vi "csm_lumikki_instron_creep_poller.vi"() -> ()   [LabVIEW 2009]
doc: "This is the sample data playback waveform and data logging example program. Sample data points are generated using MX Sample Data Array Generator.vi. You will need to replace this VI with your own code. New sample data is sent to the controller each time a status message is recieved from the controller that the next random buffer is running.\nThis program also shows you how to use Active X events. These are used to notify the program when a data buffer is ready for collection and when to load a new buffer of sample data points. Two separate event queues are used: one for data logging and the other for general status, such as when a sample data point buffer can be sent to the controller. Each event handler must run in parallel loops as execution passes to MX Handle Status Change Event.vi and MX Handle Data Ready Event.vi and will not come out of them until an event is received from the console program. When modifiying this example for your own use you may want to setup a third loop to be doing other processing, or you could add code to manipulate the data buffer in the data monitoring loop."
panel:
  in  "Maximum Value":dbl[](array[numeric]) format="%.2f"
  out "Units Strings":string[](array[string])
  in  "Control Modes":u16[](array[ring])=[0, 0, 0, 0] items=["Channel 1", "Channel 2", "Channel 3", "Channel 4"]
  in  "Number of Columns":i32[](array[numeric])
  in  "Interval/Buffer Parameters":T1={"Sample interval - ms (2)"=2.0, "Buffer Length (1000)"=1000, "No. of Buffers (0)"=0} {"Sample interval - ms (2)" min=0.2 format="%.1f"}
  in  "Column Types":i32[][](array[ring])=[[0, 0, 0, 0, 0, 0, 0, 0]] items=["Feedback", "Direct Auxillary"]
  in  "Column Channels":i32[][](array[numeric])=[[1, 1, 1, 1, 1, 1, 1, 1]] min=0 max=200
  in  "Start/Stop":bool
  in  "Axis Selector":i32[](listbox)
  # "Axis 1\nAxis 2\nAxis 3\nAxis 4"
  # "Axis 1\nAxis 2\nAxis 3\nAxis 4"
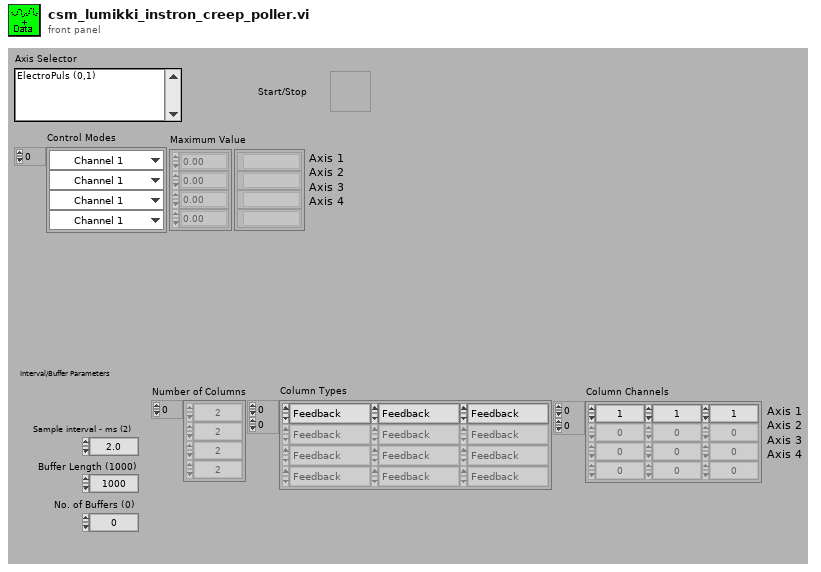
[diagram p1: front panel]
types:
  T1 = cluster{"Sample interval - ms (2)":dbl, "Buffer Length (1000)":i32, "No. of Buffers (0)":i32}
  T2 = cluster{"Name":string, "Type":i32, "SI Full Scale":dbl, "Full Scale":dbl, "Units String":string, "Display Format":string, "Gauge Length":dbl}[][]
  T3 = cluster{"Device ID":i32, "Device Name":string, "Device Type":i32}[]
  T4 = cluster{"Data Sample Format (0)":i8, "Loop code (2)":i8, "Target Amplitude (32767)":i16, "Playback rate":dbl, "Playback Scale":dbl[], "Envelope Ramp Rate":dbl, "Filter Order (0)":i8, "Filter Type (0)":i8, "Filter Bandwidth":dbl}
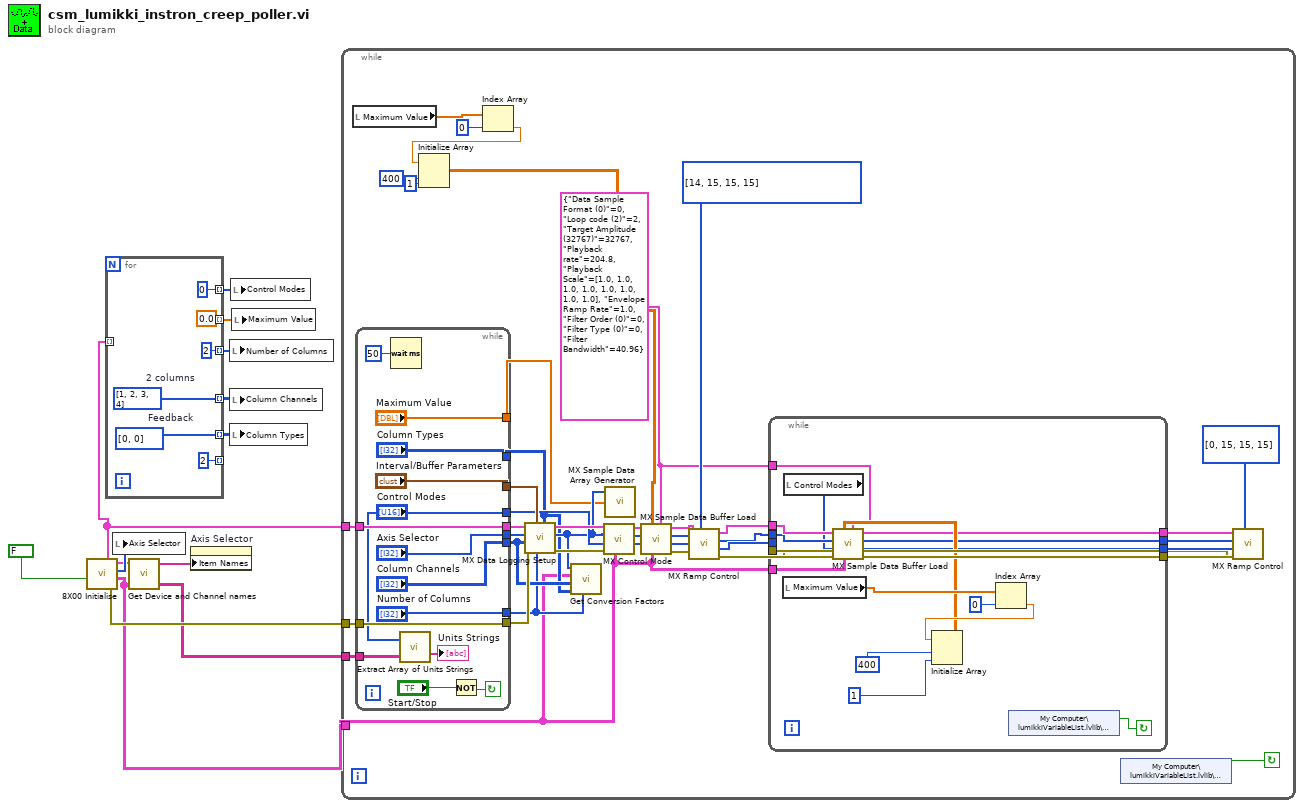
[diagram p0: block diagram]
diagram:
  n1 = call "8X00 Initialise.vi"("Reset?"=FALSE ("Reset")) -> ("error out"=w11:errorcluster, "Channel Data"=w10:T2, "Axis Selector"=w8:i32[], "Axis Information"=w1:T3)  [unwired: 3 in]
  n2 = for {
    tunnel: [w18] -> w6 mode=indexing
    tunnel: [w17] -> w5 mode=indexing
    tunnel: [2] -> _ mode=indexing
    tunnel: [2] -> w4 mode=indexing
    tunnel: [0.0] -> w3 mode=indexing
    tunnel: [0] -> w2 mode=indexing
    tunnel: w1 -> [_] mode=indexing
    w17 = i32[] [0, 0]  # Feedback
    w18 = i32[] [1, 2, 3, 4]  # 2 columns
  }
  n3 = local write "Axis Selector"(w8) -> ()
  n4 = call "Get Device and Channel names.vi"("Axis Information"=w1, "Channel Data"=w10) -> ("Device Names"=w12:string[], "Units Strings"=w9:string[][])  [unwired: 1 out]
  n5 = property on="Axis Selector" class="ListBox (strict)"("Item Names"=w12) -> ()  [unwired: 2 in, 2 out]
  n6 = local write "Number of Columns"(w4) -> ()
  n7 = local write "Column Channels"(w6) -> ()
  n8 = local write "Column Types"(w5) -> ()
  n9 = local write "Control Modes"(w2) -> ()
  n10 = local write "Maximum Value"(w3) -> ()
  n11 = while {
    tunnel: w9 -> [w42]
    tunnel: w10 -> [w20]
    tunnel: w1 -> [w54]
    tunnel: w11 -> [w57]
    stop <- w19 continue-if-true
    w30 = u16[] [0, 15, 15, 15] items=["Stop", "Start or continue", "Hold", "Continue", "Return ramp to set level at fixed rate", "Reserved", "Reserved", "Start Random without demand hold", "Start Random with demand hold", "Prepare Random Start without demand hold", "Prepare Random Start with demand hold", "Unslave", "Reserved", "Reserved", "Start Sample Data Playback or Resume", "Prepare for Start of Sample Data", "Reserved", "Reserved", "Resume Playback", "Start an electromechanical frame return"] ("Ramp Control")
    w21 = T4 {"Data Sample Format (0)"=0, "Loop code (2)"=2, "Target Amplitude (32767)"=32767, "Playback rate"=204.8, "Playback Scale"=[1.0, 1.0, 1.0, 1.0, 1.0, 1.0, 1.0, 1.0], "Envelope Ramp Rate"=1.0, "Filter Order (0)"=0, "Filter Type (0)"=0, "Filter Bandwidth"=40.96} ("Sample Data Playback Definition")
    w38 = u16[] [14, 15, 15, 15] items=["Stop", "Start or continue", "Hold", "Continue", "Return ramp to set level at fixed rate", "Reserved", "Reserved", "Start Random without demand hold", "Start Random with demand hold", "Prepare Random Start without demand hold", "Prepare Random Start with demand hold", "Unslave", "Reserved", "Reserved", "Start Sample Data Playback or Resume", "Prepare for Start of Sample Data", "Reserved", "Reserved", "Resume Playback"] ("Ramp Control")
    n12 = local read "Maximum Value"() -> (w34:dbl[])
    n13 = while {
      tunnel: ["Maximum Value"] -> w40
      tunnel: w42 -> [w79]
      tunnel: ["Control Modes"] -> w43
      tunnel: ["Number of Columns"] -> w52
      tunnel: ["Interval/Buffer Parameters"] -> w55
      tunnel: ["Column Types"] -> w37
      tunnel: [w87] -> w56
      tunnel: w57 -> [w87]
      tunnel: ["Column Channels"] -> w53
      tunnel: ["Axis Selector"] -> w58
      tunnel: [w90] -> w59
      tunnel: w54 -> [w90]
      stop <- w86 continue-if-true
      n14 = Wait (ms)(milliseconds to wait=u32 50) -> ()  [unwired: 1 out]
      n15 = call "Extract Array of Units Strings.vi"("Axes Units Strings"=w79, "Control Modes"="Control Modes") -> ("Units Strings"=→"Units Strings":string[])
      n16 = Not(x="Start/Stop") -> (.not. x?=w86:bool)
    }
    n17 = Index Array(array=w34, index=0) -> (element=w33:dbl)
    n18 = Initialize Array(w33, 400 ("dimension size"), 1 ("dimension size")) -> (w31:dbl[][])
    n19 = call "MX Data Logging Setup.vi"("Column Types"=w37, "Number of Columns"=w52, "Interval/Buffer Parameters"=w55, "error in (no error)"=w56, "Column Channels"=w53, "Axis Selector"=w58, "Axis Information"=w59) -> ("error out"=w48:errorcluster, "Axis Selector copy"=w41:i32[], "Axis Information out"=w47:T3)  [unwired: 1 out]
    n20 = call "Get Conversion Factors.vi"("Axis Selector"=w41, "Channel Data"=w20, "Column Channels"=w53, "Column Types"=w37, "Number of Columns"=w52) -> ()  [unwired: 1 out]
    n21 = call "MX Control Mode.vi"("Channel Data"=w20, "error in (no error)"=w48, "Control Modes"=w43, "Axis Selector"=w41, "Axis Information"=w47) -> ("Control Modes out"=w44:u16[], "Axis Selector out"=w45:i32[], "Axis Information out"=w46:T3)  [unwired: 1 in, 1 out]
    n22 = call "MX Sample Data Array Generator.vi"("Maximum Value"=w40, "Axis Selector"=w41) -> ()  [unwired: 1 in, 1 out]
    n23 = call "MX Sample Data Buffer Load.vi"("Sample Data Playback Definition"=w21, "Channel Data"=w20, "Sample Data"=w31, "Channels In"=w44, "Axis Selector In"=w45, "Axis Information In"=w46) -> ("error out"=w49:errorcluster, "Channels Out"=w39:u16[], "Axis Selector Out"=w50:i32[], "Axis Information Out"=w51:T3)  [unwired: 2 in]
    n24 = call "MX Ramp Control.vi"("Ramp Control"=w38, "error in (no error)"=w49, "Channels In"=w39, "Axis Selector In"=w50, "Axis Information In"=w51) -> ("error out"=w23:errorcluster, "Channels Out"=w25:u16[], "Axis Selector Out"=w24:i32[], "Axis Information Out"=w22:T3)  [unwired: 2 in]
    n25 = while {
      tunnel: w22 -> [w72]
      tunnel: w24 -> [w71]
      tunnel: w25 -> [_]
      tunnel: w23 -> [w70]
      tunnel: [w67] -> w29
      tunnel: [w66] -> w28
      tunnel: [w65] -> w27
      tunnel: [w64] -> w26
      tunnel: w21 -> [w62]
      tunnel: w20 -> [w61]
      stop <- w60 continue-if-true
      n26 = local read "Maximum Value"() -> (w69:dbl[])
      n27 = local read "Control Modes"() -> (w63:u16[])
      n28 = Index Array(array=w69, index=0) -> (element=w74:dbl)
      n29 = Initialize Array(w74, 400 ("dimension size"), 1 ("dimension size")) -> (w68:dbl[][])
      n30 = call "MX Sample Data Buffer Load.vi"("Sample Data Playback Definition"=w62, "Channel Data"=w61, "Sample Data"=w68, "error in (no error)"=w70, "Channels In"=w63, "Axis Selector In"=w71, "Axis Information In"=w72) -> ("error out"=w64:errorcluster, "Channels Out"=w65:u16[], "Axis Selector Out"=w66:i32[], "Axis Information Out"=w67:T3)  [unwired: 1 in]
      n31 = shared-variable "My Computer\\lumikkiVariableList.lvlib\\creepRunning"() -> (w60:bool)  [unwired: 1 in, 1 out]
    }
    n32 = shared-variable "My Computer\\lumikkiVariableList.lvlib\\creepRunning"() -> (w19:bool)  [unwired: 1 in, 1 out]
    n33 = call "MX Ramp Control.vi"("Ramp Control"=w30, "error in (no error)"=w26, "Channels In"=w27, "Axis Selector In"=w28, "Axis Information In"=w29) -> ()  [unwired: 2 in, 4 out]
  }
